vi "new method hmmm.vi"() -> ()   [LabVIEW 2010]
uses:
  <vilib>/Analysis/baseanly.llb/Real A x B.vi
  <vilib>/Analysis/baseanly.llb/A x Vector.vi
  <vilib>/Analysis/NI_AALBase.lvlib
panel:
  out "Cenetered":dbl[][](array[numeric])
  out "Center":dbl[](array[numeric])
  out "System Waveform Chart":dbl(graph)
  out "x+y":i32
  out "Array 2":cluster{dbl, dbl, dbl, dbl}[](array[cluster])
  out "Array":dbl[][][](array[numeric])
  out "max index(es) 2":i32[](array[numeric])
  out "max index(es)":i32[](array[numeric])
  out "max value":dbl
  out "result":dbl
  out "Box Z":dbl
  out "Box Y":dbl
  out "Box X":dbl
  out "Rotated":dbl[][](array[numeric])
  in  "Theta 3":dbl(slide)=90.0 scale=0.0..45.0
  in  "Theta 2":dbl(slide)=90.0 scale=0.0..90.0
  in  "Theta":dbl(slide)=90.0 scale=0.0..90.0
  in  "Corners":dbl[][](array[numeric])
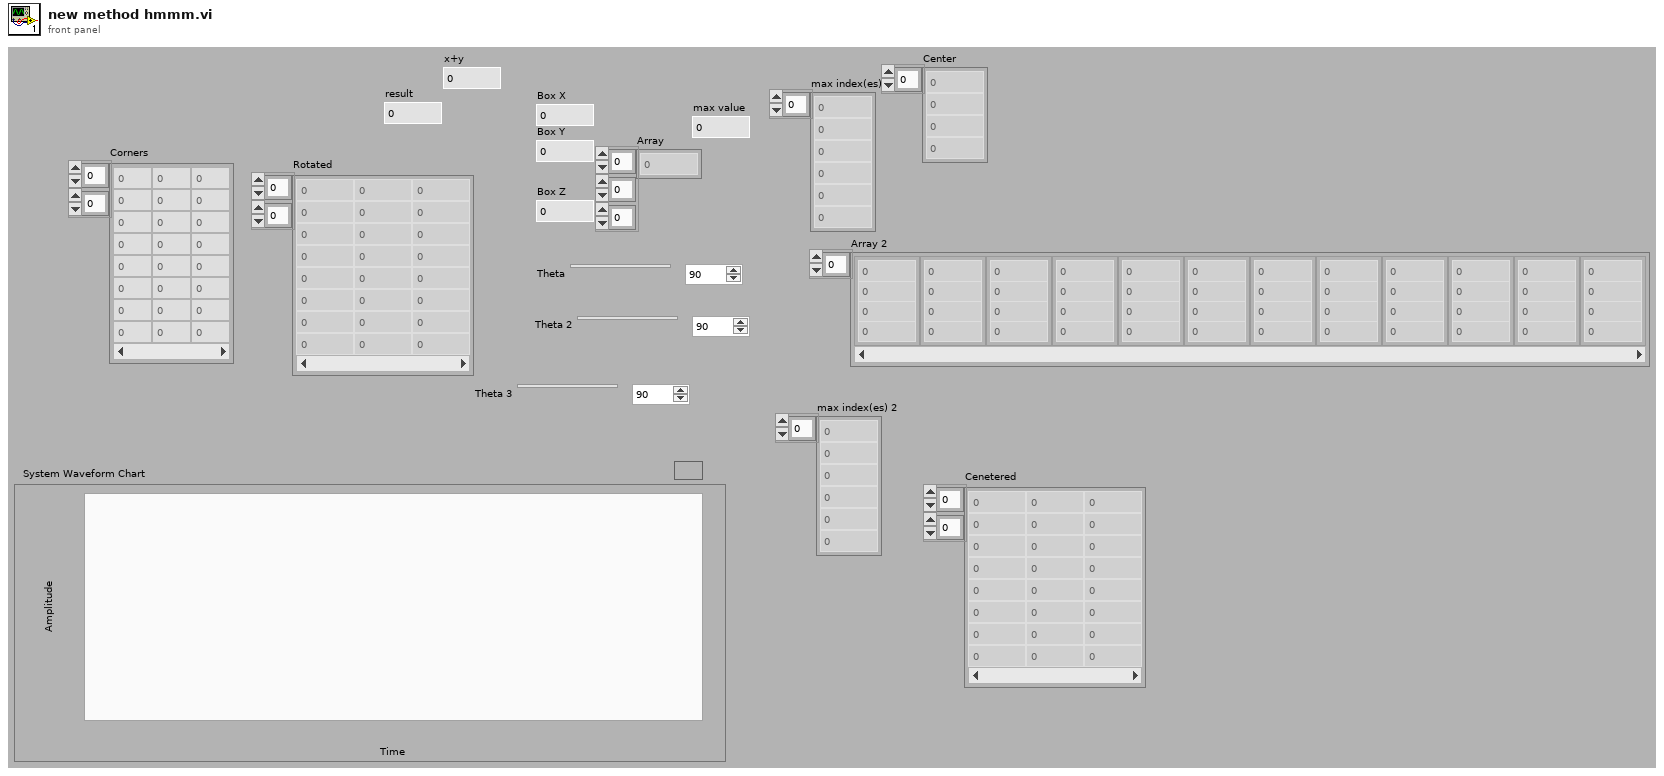
[diagram p1: front panel]
types:
  T1 = typedef "NI_Matrix.lvlib/RealMatrix.ctl" = dbl[][]
  T2 = cluster{dbl, "Theta":dbl, "Theta 2":dbl, "Theta 3":dbl}
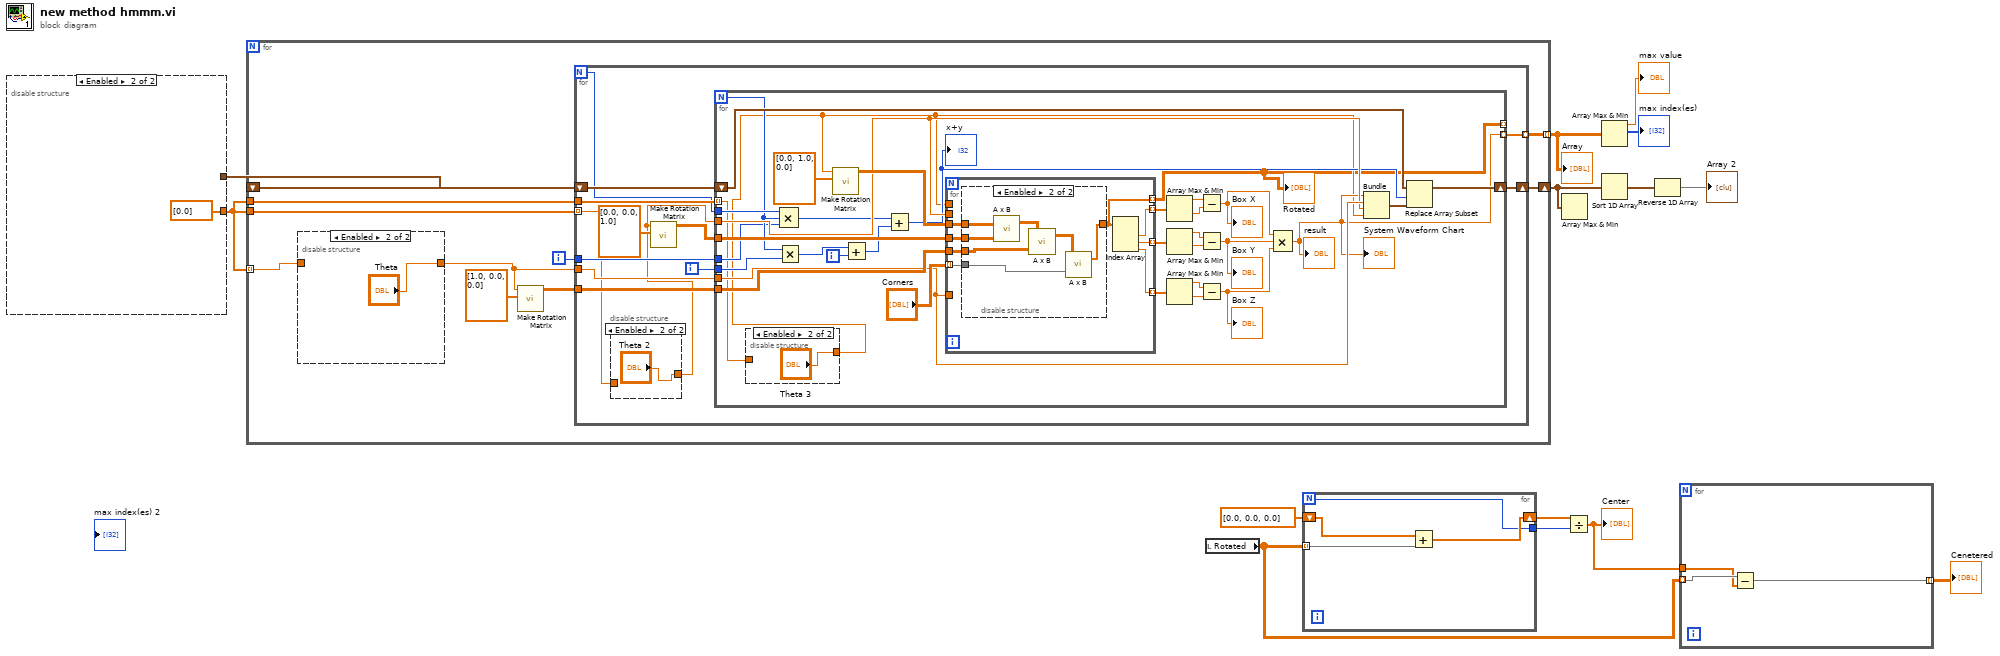
[diagram p0: block diagram]
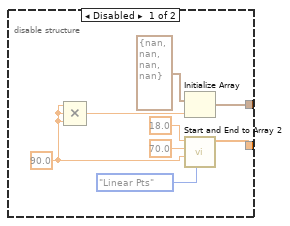
[diagram p2: hidden frame]
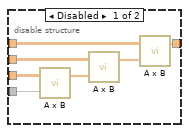
[diagram p6: hidden frame]
diagram:
  n1 = disable-structure shown="Enabled" {
    disable-tunnel: [w19 dbl[] [0.0] ("Array")] -> w14
    disable-tunnel: [w15 _] -> w10
    frame Disabled {
      w17 = 90.0 ("Step or # Pts")
      n2 = Compound Arithmetic op=MULTIPLY(w17, w17, w17) -> (w16:dbl)
      n3 = Initialize Array(cluster{dbl, dbl, dbl, dbl} {nan, nan, nan, nan}, w16) -> (w15:cluster{dbl, dbl, dbl, dbl}[])
      n4 = call "Start and End to Array 2.vi"("Sweep Style"=enum16{"Linear Step", "Linear Pts", "Log Pts"}."Linear Pts", "Step or # Pts"=w17, "End"=70.0, "Start"=18.0) -> ("Array"=w19:dbl[])  [unwired: 7 in]
    }
    frame Enabled {
    }
  }
  n5 = for {
    tunnel: w14 -> [w25] mode=indexing
    tunnel: w14 -> [w33]
    tunnel: w14 -> [w32]
    tunnel: [w31] -> w13 mode=indexing
    shift-right: [w28] -> w7
    shift-left: w10 -> [w27]
    i -> [w26]
    n6 = disable-structure shown="Enabled" {
      disable-tunnel: [w34 "Theta"] -> w24
      disable-tunnel: w25 -> [w34 _]
      frame Disabled {
      }
      frame Enabled {
      }
    }
    n7 = call "Make Rotation Matrix.vi"("Rotation Axis"=dbl[] [1.0, 0.0, 0.0], "Rotation Angle (Degree)"=w24) -> ("Rotation Matrix"=w29:T1)  [unwired: 9 in]
    n8 = for {
      N -> [w38]
      tunnel: w24 -> [w48]
      tunnel: w33 -> [w36] mode=indexing
      tunnel: w32 -> [w47]
      tunnel: [w46] -> w31 mode=indexing
      tunnel: w29 -> [w45]
      shift-right: [w42] -> w28
      shift-left: w27 -> [w41]
      tunnel: w26 -> [w39]
      i -> [w40]
      n9 = disable-structure shown="Enabled" {
        disable-tunnel: [w49 "Theta 2"] -> w37
        disable-tunnel: w36 -> [w49 _]
        frame Disabled {
        }
        frame Enabled {
        }
      }
      n10 = call "Make Rotation Matrix.vi"("Rotation Axis"=dbl[] [0.0, 0.0, 1.0], "Rotation Angle (Degree)"=w37) -> ("Rotation Matrix"=w43:T1)  [unwired: 9 in]
      n11 = for {
        N -> [w58]
        tunnel: [w51] -> _ mode=indexing
        tunnel: w48 -> [w68]
        tunnel: w37 -> [w67]
        tunnel: w47 -> [w52] mode=indexing
        tunnel: [w54] -> w46 mode=indexing
        tunnel: w45 -> [w72]
        tunnel: w43 -> [w71]
        shift-right: [w64] -> w42
        shift-left: w41 -> [w65]
        tunnel: w40 -> [w62]
        tunnel: w39 -> [w57]
        tunnel: w38 -> [w59]
        i -> [w63]
        n12 = disable-structure shown="Enabled" {
          disable-tunnel: [w86 "Theta 3"] -> w53
          disable-tunnel: w52 -> [w86 _]
          frame Disabled {
          }
          frame Enabled {
          }
        }
        n13 = Multiply(x=w58, y=w62) -> (x*y=w61:i32)
        n14 = Compound Arithmetic op=MULTIPLY(w59, w58, w57) -> (w56:i32)
        n15 = call "Make Rotation Matrix.vi"("Rotation Axis"=dbl[] [0.0, 1.0, 0.0], "Rotation Angle (Degree)"=w53) -> ("Rotation Matrix"=w69:T1)  [unwired: 9 in]
        n16 = Add(x=w61, y=w63) -> (x+y=w60:i32)
        n17 = Add(x=w56, y=w60) -> (x+y=w55:i32)
        "x+y" <- w55
        n18 = for {
          tunnel: "Corners" -> [w95] mode=indexing
          tunnel: [w94] -> w51 mode=indexing
          tunnel: [w93] -> w75 mode=indexing
          tunnel: [w92] -> w74 mode=indexing
          tunnel: [w91] -> w73 mode=indexing
          tunnel: w68 -> [_]
          tunnel: w67 -> [_]
          tunnel: w53 -> [_]
          tunnel: w72 -> [w90]
          tunnel: w71 -> [w89]
          tunnel: w69 -> [w88]
          n19 = disable-structure shown="Enabled" {
            disable-tunnel: w95 -> [w102 w104]
            disable-tunnel: [w99 w103] -> w94
            disable-tunnel: w90 -> [w98 w106]
            disable-tunnel: w89 -> [w97 w108]
            disable-tunnel: w88 -> [w96 w109]
            frame Disabled {
              n20 = call-poly <vilib>:"A x B.vi"("Vector"=w102, "A"=w98) -> ("A x Vector"=w101:dbl[])  [unwired: 1 out]
              n21 = call-poly <vilib>:"A x B.vi"("Vector"=w101, "A"=w97) -> ("A x Vector"=w100:dbl[])  [unwired: 1 out]
              n22 = call-poly <vilib>:"A x B.vi"("Vector"=w100, "A"=w96) -> ("A x Vector"=w99:dbl[])  [unwired: 1 out]
            }
            frame Enabled {
              n23 = call-poly <vilib>:"A x B.vi"("B"=w108, "A"=w109) -> ("A x B"=w107:T1)  [unwired: 1 out]
              n24 = call-poly <vilib>:"A x B.vi"("B"=w106, "A"=w107) -> ("A x B"=w105:T1)  [unwired: 1 out]
              n25 = call-poly <vilib>:"A x B.vi"("Vector"=w104, "A"=w105) -> ("A x Vector"=w103:dbl[])  [unwired: 1 out]
            }
          }
          n26 = Index Array(array=w94) -> (element #1=w93:dbl, element #2=w92:dbl, element #3=w91:dbl)  [unwired: 3 in]
        }
        "Rotated" <- w51
        n27 = Array Max & Min(array=w75) -> (max value=w76:dbl, min value=w77:dbl)  [unwired: 2 out]
        n28 = Array Max & Min(array=w74) -> (max value=w79:dbl, min value=w78:dbl)  [unwired: 2 out]
        n29 = Array Max & Min(array=w73) -> (max value=w80:dbl, min value=w81:dbl)  [unwired: 2 out]
        n30 = Subtract(x=w76, y=w77) -> (x-y=w82:dbl)
        "Box X" <- w82
        n31 = Subtract(x=w79, y=w78) -> (x-y=w83:dbl)
        "Box Y" <- w83
        n32 = Subtract(x=w80, y=w81) -> (x-y=w84:dbl)
        "Box Z" <- w84
        n33 = Compound Arithmetic op=MULTIPLY(w82, w83, w84) -> (w54:dbl)
        "result" <- w54
        "System Waveform Chart" <- w54
        n34 = Bundle(w54, "Theta"=w68, "Theta 2"=w67, "Theta 3"=w53) -> (w66:T2)  [unwired: 1 in]
        n35 = Replace Array Subset(array=w65, new element=w66, index=w55) -> (w64:cluster{dbl, dbl, dbl, dbl}[])
      }
    }
  }
  "Array" <- w13
  n36 = local read "Rotated"() -> (w3:dbl[][])
  n37 = for {
    N -> [w110]
    tunnel: w3 -> [w113] mode=indexing
    shift-right: [w112] -> w5
    shift-left: dbl[] [0.0, 0.0, 0.0] -> [w111]
    tunnel: [w110] -> w4
    n38 = Add(x=w111, y=w113) -> (x+y=w112:dbl[])
  }
  n39 = Array Max & Min(array=w7) -> ()  [unwired: 4 out]
  n40 = Divide(x=w5, y=w4) -> (x/y=w2:dbl[])
  "Center" <- w2
  n41 = Array Max & Min(array=w13) -> (max value=→"max value":dbl, max index (indices)=→"max index(es)":i32[])  [unwired: 2 out]
  n42 = Sort 1D Array(array=w7) -> (sorted array=w9:cluster{dbl, dbl, dbl, dbl}[])
  n43 = Reverse 1D Array(array=w9) -> (reversed array=→"Array 2":cluster{dbl, dbl, dbl, dbl}[])
  n44 = for {
    tunnel: w3 -> [w116] mode=indexing
    tunnel: w2 -> [w115]
    tunnel: [w114] -> w1 mode=indexing
    n45 = Subtract(x=w116, y=w115) -> (x-y=w114:dbl[])
  }
  "Cenetered" <- w1
